vi "Actor Core.vi"(8 "error in":errorcluster, 11 "Simulated Entry Console Actor in":refnum<class "Simulated Entry Console Actor.lvclass">) -> (0 "error out":errorcluster, 3 "Actor out":refnum<class "Actor.lvclass">)   [LabVIEW 2019, in "Simulated Entry Console Actor.lvlib" / "Simulated Entry Console Actor.lvclass"]
doc: "(<B>Filename</B>: Actor Framework.lvlib:Actor.lvclass:Actor Core.vi)\n\nReceives messages to the actor, reacts to them, and initiates any error handling that may shut the actor down.\n\nDescendant classes may override this VI to append parallel tasks for the actor to complete while it handles messages. Overrides use the Call Parent Method node."
uses:
  Simulated Entry Console Actor.lvclass
  <vilib>/ActorFramework/Stop Msg/Stop Msg.lvclass
  <vilib>/ActorFramework/Actor/Actor.lvclass
  Car Wash Controller Actor/Car Wash Controller Actor Messages/Set State Msg/Set State Msg.lvclass
  C:/Workspace/CLA/Carwasher AF/Abstract Entry Console Actor/Abstract Entry Console Actor/Entry Console Actor.lvclass
  C:/Program Files (x86)/National Instruments/LabVIEW 2019/vi.lib/ActorFramework/Actor/Actor.lvclass
  Car Wash Controller Actor/Car Wash Controller Actor/State -Enum.ctl
  Car Wash Controller Actor/Car Wash Controller Actor/Car Wash Controller Actor.lvclass
  Abstract Entry Console Actor/Abstract Entry Console Actor/Entry Console Actor.lvclass
  Wash steps selection -Buttons.ctl
  Car Wash Controller Actor/Car Wash Controller Actor Messages/Set Display Wash Step from User Console Msg/Set Display Wash Step from User Console Msg.lvclass
panel:
  in  "Start":bool
  in  "Wash steps selection buttons":T1
  # "Entry Console"
  # "UI1."
  # "UI2."
  # "UI2A4."
  # "WS2A."
  # "UI2B."
  # "UI2B1."
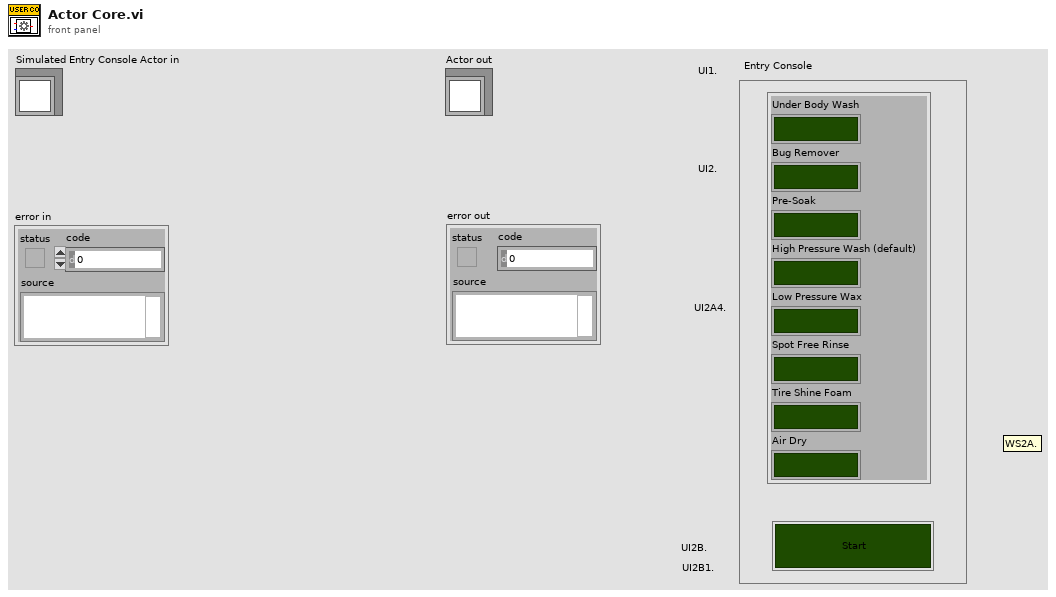
[diagram p1: front panel]
types:
  T1 = typedef "Simulated Entry Console Actor.lvlib/Simulated Entry Console Actor.lvclass/Wash steps selection -Buttons.ctl" = cluster{"Under Body Wash":bool, "Bug Remover":bool, "Pre-Soak":bool, "High Pressure Wash (default)":bool, "Low Pressure Wax":bool, "Spot Free Rinse":bool, "Tire Shine Foam":bool, "Air Dry":bool}
  T2 = typedef "Car Wash Controller Actor.lvlib/Car Wash Controller Actor.lvclass/State -Enum.ctl" = enum16{"Initial", "Wait for Start", "Start", "Wait for Vehicle Position", "Wash Step Execution", "Wash Step/Cycle Completion", "Wash Exit", "Wash Abort/Terminate"}
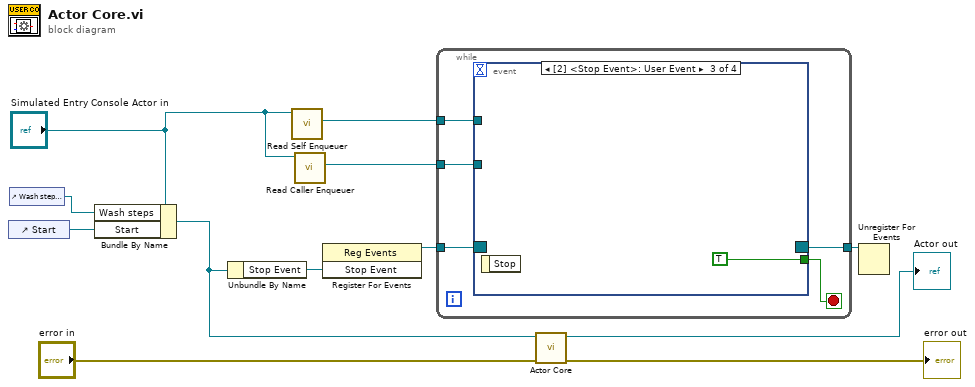
[diagram p0: block diagram]
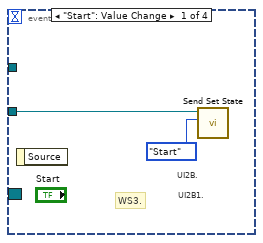
[diagram p2: hidden frame]
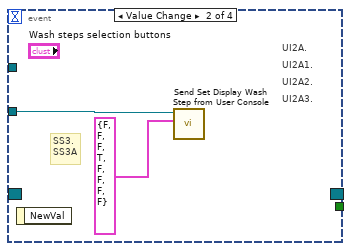
[diagram p3: hidden frame]
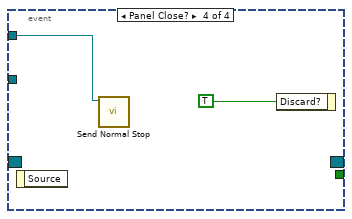
[diagram p4: hidden frame]
diagram:
  n1 = control-ref of="Start"() -> (w8:refnum<vi>)
  n2 = control-ref of="Wash steps selection buttons"() -> (w9:refnum<vi>)
  n3 = Bundle By Name(cluster="Simulated Entry Console Actor in", "Wash steps"=w9, "Start"=w8) -> (w7:refnum<class "Simulated Entry Console Actor.lvclass">)
  n4 = Unbundle By Name(w7) -> ("Stop Event"=w6:refnum<user-event>)
  n5 = call <vilib>:"Read Self Enqueuer.vi"("Actor"="Simulated Entry Console Actor in") -> ("Self Enqueuer"=w3:refnum<class "Message Enqueuer.lvclass">)  [unwired: 10 in]
  n6 = call <vilib>:"Read Caller Enqueuer.vi"("Actor"="Simulated Entry Console Actor in") -> ("Caller Enqueuer"=w1:refnum<class "Message Enqueuer.lvclass">)  [unwired: 10 in]
  n7 = register-events(w6) -> (reference out=w5:refnum<event-registration>)  [unwired: 2 in, 1 out]
  n8 = while {
    tunnel: w5 -> [w16]
    tunnel: [w15] -> w4
    tunnel: w3 -> [w14]
    tunnel: w1 -> [w13]
    stop <- w17 stop-if-true
    n9 = event shown="[2] <Stop Event>: User Event" {
      selector: w16 -> [_ _ _ _]
      dyn-events: [_ _ _ _] -> w15
      timeout: _ -> [_ _ _ _]
      tunnel: [_ _ TRUE _] -> w17
      tunnel: w14 -> [_ _ _ w23]
      tunnel: w13 -> [w19 w21 _ _]
      event "Start": Value Change {
        # "WS3."
        # "UI2B1."
        # "UI2B."
        n10 = event-data() -> ()  [unwired: 1 in, 1 out]
        n11 = call "Send Set State.vi"("States"=State_-Enum."Start", "Message Enqueuer"=w19) -> ()  [unwired: 8 in, 2 out]
      }
      event Value Change {
        # "SS3.\nSS3A"
        # "UI2A3."
        # "UI2A2."
        # "UI2A1."
        # "UI2A."
        n12 = event-data() -> ()  [unwired: 1 in, 1 out]
        n13 = call "Send Set Display Wash Step from User Console.vi"("Wash Steps"=T1 {"Under Body Wash"=FALSE, "Bug Remover"=FALSE, "Pre-Soak"=FALSE, "High Pressure Wash (default)"=TRUE, "Low Pressure Wax"=FALSE, "Spot Free Rinse"=FALSE, "Tire Shine Foam"=FALSE, "Air Dry"=FALSE} ("Wash steps selection buttons"), "Message Enqueuer"=w21) -> ()  [unwired: 8 in, 2 out]
      }
      event User Event {
        n14 = event-data() -> ()  [unwired: 1 in, 1 out]
      }
      event Panel Close? {
        n15 = event-data() -> ()  [unwired: 1 in, 1 out]
        n16 = call <vilib>:"Send Normal Stop.vi"("Message Enqueuer"=w23) -> ()  [unwired: 10 in, 1 out]
        n17 = event-data("Discard?"=TRUE) -> ()  [unwired: 1 in, 1 out]
      }
    }
  }
  n18 = call-parent "Actor Core.vi"("error in"="error in", "Actor in"=w7) -> ("error out"=→"error out":errorcluster, "Actor out"=→"Actor out":refnum<class "Actor.lvclass">)  [unwired: 8 in]
  n19 = Unregister For Events(event registration refnum=w4) -> ()  [unwired: 1 in, 1 out]
